vi "Select channel.vi"(4 "length":i32, 6 "index":i32, 8 "err in":errorcluster, 10 "Data in":u64[][](array[numeric])) -> (0 "err out":errorcluster, 3 "output waveform":waveform(cdb), 7 "Data in size":i32[](array[numeric]))   [LabVIEW 2015, in "Monitoring_receiver.lvlib"]
uses:
  Monitoring_receiver.lvlib
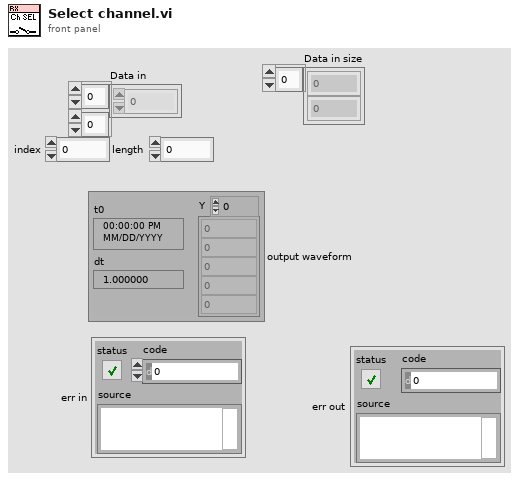
[diagram p1: front panel]
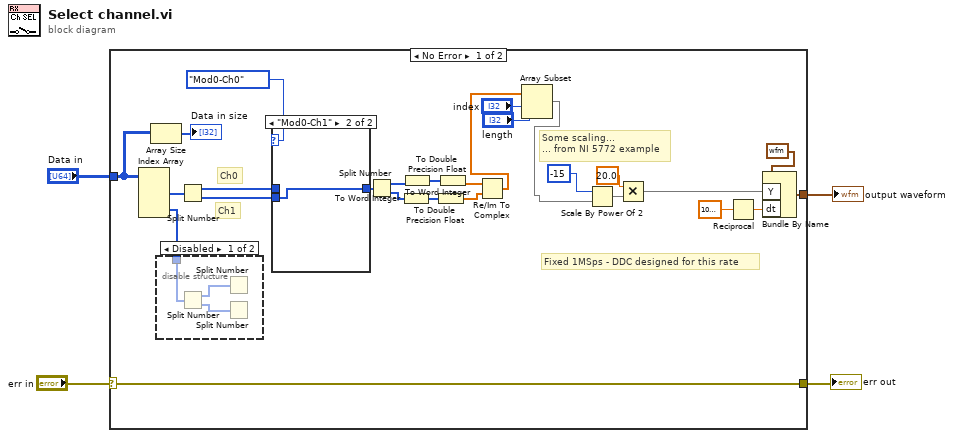
[diagram p0: block diagram]
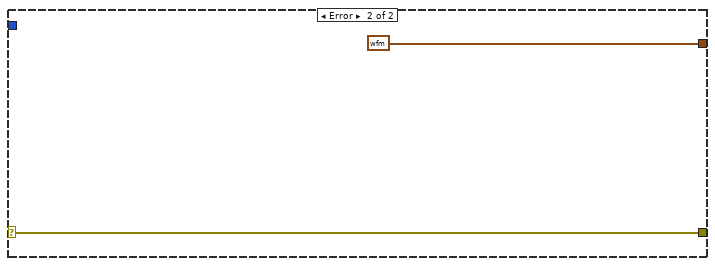
[diagram p4: hidden frame]
diagram:
  n1 = case shown="No Error" "err in" {
    selector: "err in" -> [w9 w38]
    tunnel: "Data in" -> [w28 _]
    tunnel: [w10 waveform(cdb) {"t0"=timestamp(0 s since 1904-01-01), "dt"=1.0, "Y"=[]} ("time signal")] -> w3
    tunnel: [w9 w38] -> w1
    frame No Error {
      # "Fixed 1MSps - DDC designed for this rate"
      # "Some scaling...\n... from NI 5772 example"
      # "Ch1"
      # "Ch0"
      n2 = Index Array(array=w28) -> (element #1=w30:u64[], element #2=w29:u64[])  [unwired: 4 in]
      n3 = Array Size(array=w28) -> (size(s)=→"Data in size":i32[])
      n4 = disable-structure shown="Disabled" {
        disable-tunnel: w29 -> [w34 _]
        frame Disabled {
          n5 = Split Number(x=w34) -> (hi(x)=w33:u32[], lo(x)=w32:u32[])
          n6 = Split Number(x=w33) -> ()  [unwired: 2 out]
          n7 = Split Number(x=w32) -> ()  [unwired: 2 out]
        }
        frame Enabled {
        }
      }
      n8 = Split Number(x=w30) -> (hi(x)=w23:u32[], lo(x)=w22:u32[])
      n9 = case shown="\"Mod0-Ch1\"" enum16{"Mod0-Ch0", "Mod0-Ch1"}."Mod0-Ch0" {
        tunnel: w23 -> [w35 _]
        tunnel: w22 -> [_ w36]
        tunnel: [w35 w36] -> w21
        frame "Mod0-Ch0", Default {
        }
        frame "Mod0-Ch1" {
        }
      }
      n10 = Split Number(x=w21) -> (hi(x)=w20:u16[], lo(x)=w19:u16[])
      n11 = To Word Integer(number=w19) -> (16bit integer=w17:i16[])
      n12 = To Word Integer(number=w20) -> (16bit integer=w18:i16[])
      n13 = To Double Precision Float(number=w17) -> (double precision float=w15:dbl[])
      n14 = To Double Precision Float(number=w18) -> (double precision float=w16:dbl[])
      n15 = Re/Im To Complex(1:w15, 2:w16) -> (0:w6:cdb[])
      n16 = Array Subset(array=w6, index="index", length="length") -> (w5:cdb[])
      n17 = Scale By Power Of 2(n=i16 -15, x=w5) -> (x*2^n=w26:cdb[])
      n18 = Multiply(x=20.0, y=w26) -> (x*y=w13:cdb[])
      n19 = Reciprocal(x=1000000.0) -> (1/x=w12:dbl)
      n20 = Bundle By Name(cluster=waveform(cdb) {"t0"=timestamp(0 s since 1904-01-01), "dt"=1.0, "Y"=[]} ("time signal"), "Y"=w13, "dt"=w12) -> (w10:waveform(cdb))
    }
    frame Error {
    }
  }
  "output waveform" <- w3
  "err out" <- w1
